vi "rpopup.vi"() -> ()   [LabVIEW 2014]
doc: "Target VI used in conjunction with the asynchronous call examples."
uses:
  subVI/version.vi
panel:
  in  "닫기":bool
  out "?":string="\n"
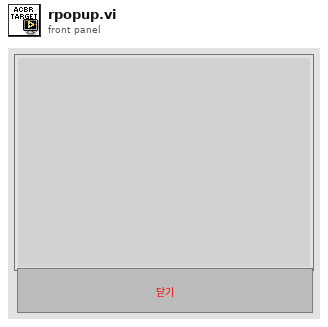
[diagram p1: front panel]
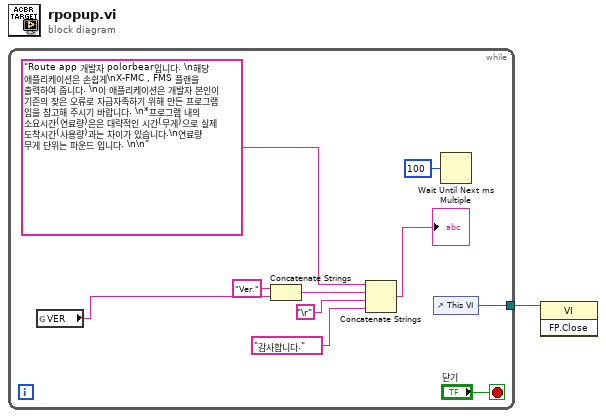
[diagram p0: block diagram]
diagram:
  n1 = while {
    tunnel: [w10] -> w1
    stop <- "닫기" stop-if-true
    n2 = global read "version.vi" "VER"() -> (w5:string)
    n3 = Concatenate Strings("Ver." ("문자열"), w5) -> (w6:string)
    n4 = Concatenate Strings("Route app 개발자 polorbear입니다. \n해당 애플리케이션은 손쉽게\nX-FMC , FMS 플랜을 출력하여 줍니다. \n이 애플리케이션은 개발자 본인이 기존의 잦은 오류로 자급자족하기 위해 만든 프로그램 임을 참고해 주시기 바랍니다. \n*프로그램 내의 소요시간(연료량)은은 대략적인 시간(무게)으로 실제 도착시간(사용량)과는 차이가 있습니다.\n연료량 무게 단위는 파운드 입니다. \n\n", w6, "\r", "감사합니다." ("문자열")) -> (→"?":string)
    n5 = control-ref of="This VI"() -> (w10:refnum<vi>)
    n6 = Wait Until Next ms Multiple(millisecond multiple=u32 100 ("ms 배수")) -> ()  [unwired: 1 out]
  }
  n7 = invoke class="VI" method="FP.Close"(reference=w1) -> ()  [unwired: 2 in, 3 out]
